vi "Simple Client.vi"(8 "error in (no error)":errorcluster, 9 "Data":variant, 10 "Command":string, 11 "RemoteControl in":refnum<class "RemoteControl.lvclass">) -> (0 "error out":errorcluster, 1 "Data out":variant, 2 "Command out":string, 3 "RemoteControl out":refnum<class "RemoteControl.lvclass">)   [LabVIEW 2016, in "RemoteControl.lvclass"]
uses:
  RemoteControl.lvclass
panel:
  out "# reads":i32
  out "execution time (ms)":u32
  # "Simple Client"
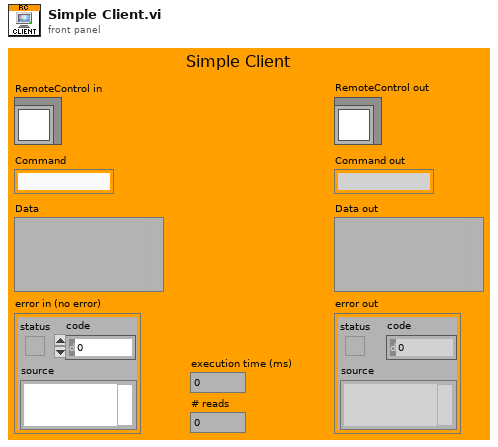
[diagram p1: front panel]
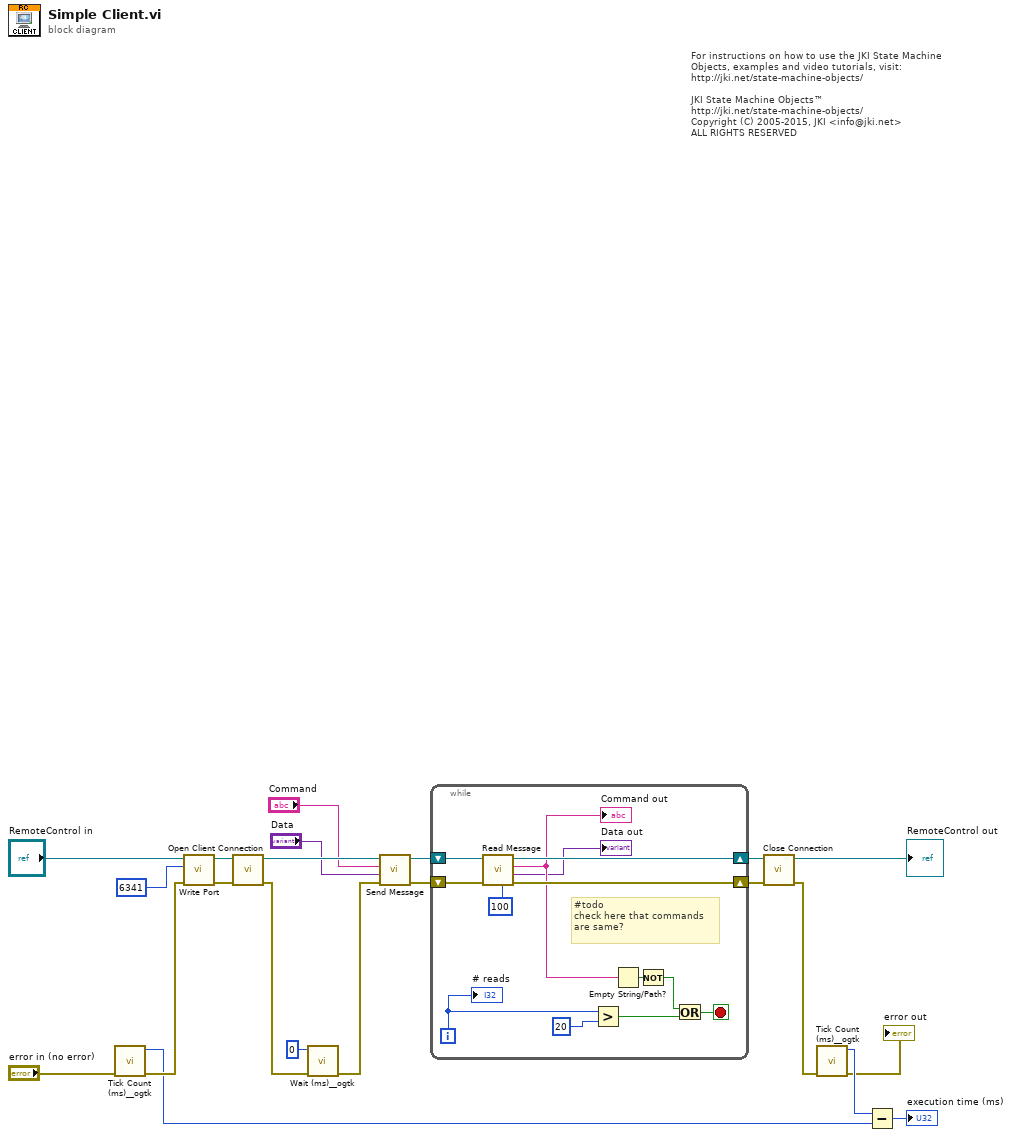
[diagram p0: block diagram]
diagram:
  # "For instructions on how to use the JKI State Machine Objects, examples and video tutorials, visit:\nhttp://jki.net/state-machine-objects/\n\nJKI State Machine Objects™\nhttp://jki.net/state-machine-objects/\nCopyright (C) 2005-2015, JKI <info@jki.net>\nALL RIGHTS RESERVED"
  n1 = call <userlib>:"Tick Count (ms)__ogtk.vi"("error in (no error)"="error in (no error)") -> ("error out"=w22:errorcluster, "millisecond timer value"=w18:u32)  [unwired: 9 in]
  n2 = call-dynamic "Write Port.vi"("error in (no error)"=w22, "Port"=u32 6341, "RemoteControl in"="RemoteControl in") -> ("error out"=w11:errorcluster, "RemoteControl out"=w12:refnum<class "RemoteControl.lvclass">)  [unwired: 7 in]
  n3 = call-dynamic "Open Client Connection.vi"("error in (no error)"=w11, "RemoteControl in"=w12) -> ("error out"=w5:errorcluster, "RemoteControl out"=w13:refnum<class "RemoteControl.lvclass">)  [unwired: 8 in]
  n4 = call <userlib>:"Wait (ms)__ogtk.vi"("error in (no error)"=w5, "milliseconds to wait"=u32 0) -> ("error out"=w6:errorcluster)  [unwired: 8 in, 1 out]
  n5 = call-dynamic "Send Message.vi"("error in (no error)"=w6, "Data"="Data", "Command"="Command", "RemoteControl in"=w13) -> ("error out"=w14:errorcluster, "RemoteControl out"=w15:refnum<class "RemoteControl.lvclass">)  [unwired: 6 in]
  n6 = while {
    shift-right: [w35] -> w17
    shift-left: w15 -> [w33]
    shift-right: [w34] -> w16
    shift-left: w14 -> [w32]
    i -> [w28]
    stop <- w29 stop-if-true
    # "#todo\ncheck here that commands\nare same?"
    n7 = call-dynamic "Read Message.vi"("timeout in ms (100)"=100, "error in (no error)"=w32, "RemoteControl in"=w33) -> ("error out"=w34:errorcluster, "Data"=→"Data out":variant, "Command"=w25:string, "RemoteControl out"=w35:refnum<class "RemoteControl.lvclass">)  [unwired: 4 in, 1 out]
    "Command out" <- w25
    n8 = Greater?(x=w28, y=20) -> (0:w27:bool)
    n9 = Empty String/Path?(string/path=w25) -> (empty?=w30:bool)
    n10 = Not(x=w30) -> (.not. x?=w23:bool)
    n11 = Or(x=w23, y=w27) -> (x .or. y?=w29:bool)
    "# reads" <- w28
  }
  n12 = call-dynamic "Close Connection.vi"("error in (no error)"=w16, "RemoteControl in"=w17) -> ("error out"=w4:errorcluster, "RemoteControl out"=→"RemoteControl out":refnum<class "RemoteControl.lvclass">)  [unwired: 8 in]
  n13 = call <userlib>:"Tick Count (ms)__ogtk.vi"("error in (no error)"=w4) -> ("error out"=→"error out":errorcluster, "millisecond timer value"=w21:u32)  [unwired: 9 in]
  n14 = Subtract(x=w21, y=w18) -> (x-y=→"execution time (ms)":u32)
